vi "sub step que.vi"(8 "error in":errorcluster, 11 "Sub step in":T1) -> (0 "error out":errorcluster, 3 "Sub step out":T1)   [LabVIEW 2014]
uses:
  Control/Sub step profiler.ctl
  <vilib>/Automated Test Systems Ltd/General Tools/Que lib/Write.vi
  <vilib>/Automated Test Systems Ltd/General Tools/Que lib/Que lib.lvlib
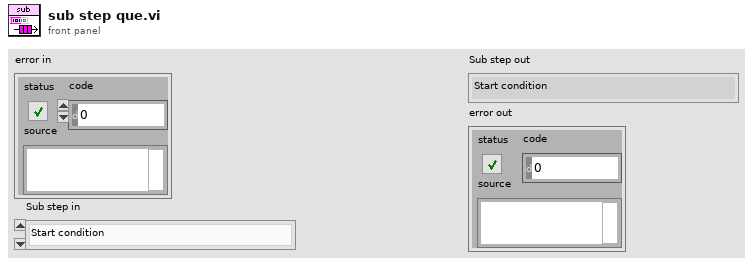
[diagram p1: front panel]
types:
  T1 = typedef "Sub step profiler.ctl" = enum16{"Start condition", "Constant condition", "End condition", "Fail", "Complete"}
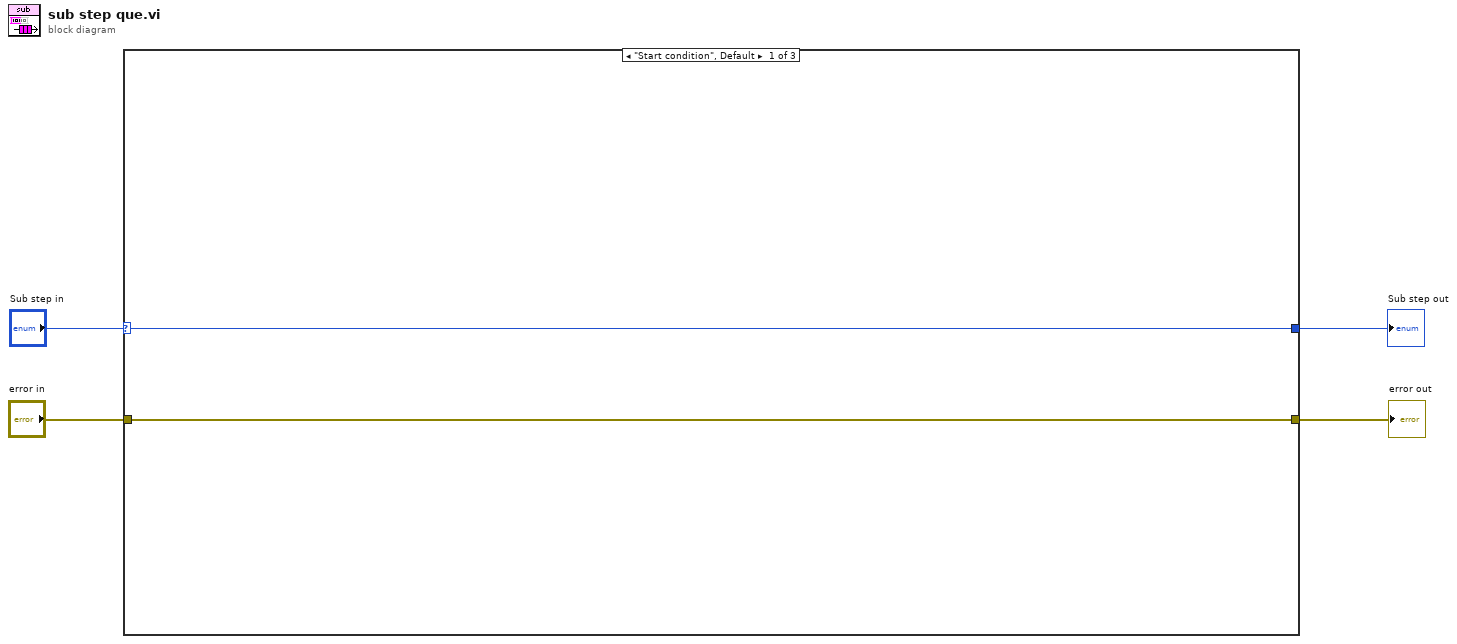
[diagram p0: block diagram]
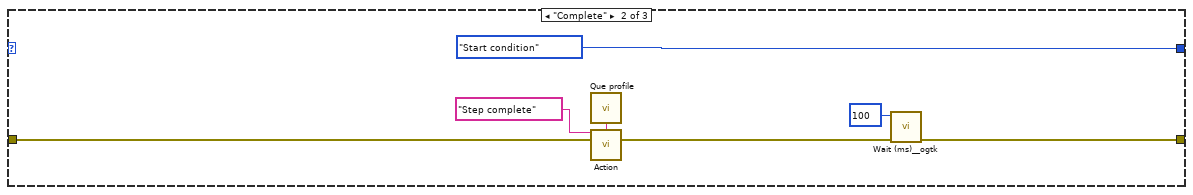
[diagram p2: hidden frame]
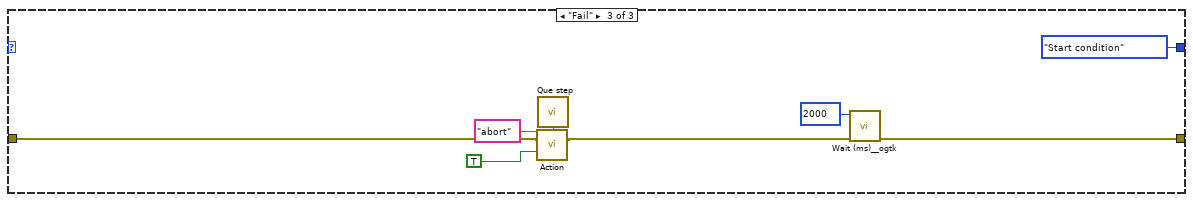
[diagram p3: hidden frame]
diagram:
  n1 = case shown="\"Start condition\", Default" "Sub step in" {
    selector: "Sub step in" -> [w5 _ _]
    tunnel: "error in" -> [w6 w9 w17]
    tunnel: [w6 w12 w20] -> w3
    tunnel: [w5 Sub_step_profiler."Start condition" ("Sub step out") Sub_step_profiler."Start condition" ("Sub step out")] -> w4
    frame "Start condition", Default {
    }
    frame "Complete" {
      n2 = call <vilib>:"Que profile.vi"() -> ("Que name"=w7:string)  [unwired: 15 in]
      n3 = call-poly <vilib>:"Action.vi"("Message"="Step complete", "Que name"=w7, "error in"=w9) -> ("error out"=w10:errorcluster)  [unwired: 12 in]
      n4 = call <userlib>:"Wait (ms)__ogtk.vi"("error in (no error)"=w10, "milliseconds to wait"=u32 100) -> ("error out"=w12:errorcluster)  [unwired: 8 in, 1 out]
    }
    frame "Fail" {
      n5 = call <vilib>:"Que step.vi"() -> ("Que name"=w15:string)  [unwired: 15 in]
      n6 = call-poly <vilib>:"Action.vi"("Message"="abort" ("Command"), "Que name"=w15, "error in"=w17, "Priority message?"=TRUE) -> ("error out"=w16:errorcluster)  [unwired: 11 in]
      n7 = call <userlib>:"Wait (ms)__ogtk.vi"("error in (no error)"=w16, "milliseconds to wait"=u32 2000) -> ("error out"=w20:errorcluster)  [unwired: 8 in, 1 out]
    }
  }
  "Sub step out" <- w4
  "error out" <- w3
